vi "class_data.vi"() -> ()   [LabVIEW 2010, in "TrajectoryAK101022Resonance.lvclass"]
uses:
  TrajectoryAK101022Resonance.lvclass
panel:
  in  "x scan segment fraction":dbl
  in  "x offset fly back fraction":dbl
  in  "x offset fly forward fraction":dbl
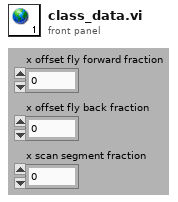
[diagram p1: front panel]
diagram:
